vi "Initialize_Array.vi"(8 "Dimensions for 2D":T1, 9 "Dimension 1D Array":i32, 10 "Value":i8, 11 "Choose Initialize Array":T2) -> (1 "Initialized Array 2D":i8[][](array[numeric]), 2 "Initialized Array 1D":i8[](array[numeric]))   [LabVIEW 2018]
uses:
  Controls/1D_2D.ctl
  Controls/Rows_Columns.ctl
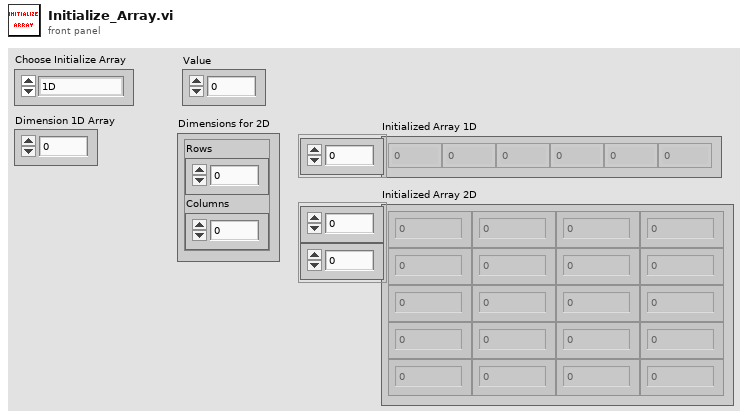
[diagram p1: front panel]
types:
  T1 = typedef "Rows_Columns.ctl" = cluster{"Rows":i32, "Columns":i32}
  T2 = typedef "1D_2D.ctl" = enum16{"1D", "2D"}
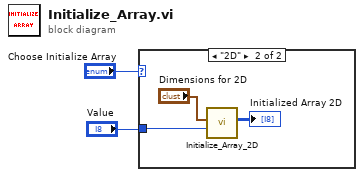
[diagram p0: block diagram]
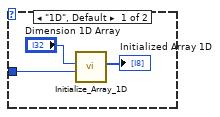
[diagram p2: hidden frame]
diagram:
  n1 = case shown="\"2D\"" "Choose Initialize Array" {
    tunnel: "Value" -> [w3 w7]
    frame "1D", Default {
      n2 = call "Initialize_Array_1D.vi"("Value"=w3, "Dimension 1D Array"="Dimension 1D Array") -> ("Initialized Array 1D"=→"Initialized Array 1D":i8[])  [unwired: 9 in]
    }
    frame "2D" {
      n3 = call "Initialize_Array_2D.vi"("Value"=w7, "Dimensions"="Dimensions for 2D") -> ("Initialized Array 2D"=→"Initialized Array 2D":i8[][])  [unwired: 9 in]
    }
  }
